vi "Obtain Motor Communication.vi"(8 "error in (no error)":errorcluster, 11 "motor name":string) -> (0 "error out":errorcluster, 1 "found?":bool, 3 "motor communication out":refnum<class "NI_Robotics_Motor Communication.lvclass">)   [LabVIEW 2017, in "NI_Robotics_Motor Communication.lvclass"]
doc: "Obtains and existing communication session for a motor."
uses:
  <vilib>/robotics/Actuation/Motor Communication/NI_Robotics_Motor Communication.lvclass
  <vilib>/robotics/Actuation/Motor Communication/FG Motor Comm Sessions Action.ctl
  <vilib>/robotics/Utilities/Generate Error.vi
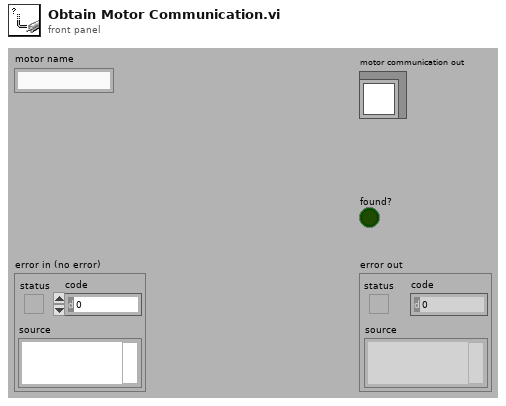
[diagram p1: front panel]
types:
  T1 = typedef "NI_Robotics_Motor Communication.lvclass/FG Motor Comm Sessions Action.ctl" = enum16{"Get", "Add", "Delete"}
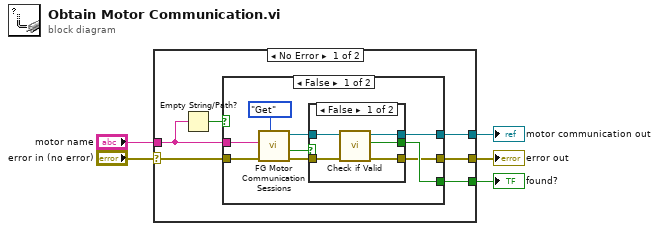
[diagram p0: block diagram]
diagram:
  n1 = case shown="No Error" "error in (no error)" {
    selector: "error in (no error)" -> [w11 w29]
    tunnel: [w9 w29] -> w4
    tunnel: [w8 _] -> w3
    tunnel: "motor name" -> [w7 _]
    tunnel: [w10 _] -> w1
    frame No Error {
      n2 = Empty String/Path?(string/path=w7) -> (empty?=w6:bool)
      n3 = case shown="False" w6 {
        tunnel: w11 -> [w19 w28]
        tunnel: [w15 _] -> w10
        tunnel: [w14 w28] -> w9
        tunnel: [w13 _] -> w8
        tunnel: w7 -> [w12 _]
        frame False {
          n4 = call <vilib>:"FG Motor Communication Sessions.vi"("action"=FG_Motor_Comm_Sessions_Action."Get", "error in (no error)"=w19, "motor name"=w12) -> ("error out"=w18:errorcluster, "failed?"=w16:bool, "motor communication out"=w17:refnum<class "NI_Robotics_Motor Communication.lvclass">)  [unwired: 6 in]
          n5 = case shown="False" w16 {
            tunnel: w17 -> [w25 w26]
            tunnel: [w24 w26] -> w13
            tunnel: w18 -> [w23 w27]
            tunnel: [w21 _] -> w15
            tunnel: [w22 w27] -> w14
            frame False {
              n6 = call <vilib>:"Check if Valid.vi"("error in (no error)"=w23, "motor communication in"=w25) -> ("error out"=w22:errorcluster, "valid?"=w21:bool, "motor communication out"=w24:refnum<class "NI_Robotics_Motor Communication.lvclass">)  [unwired: 7 in]
            }
            frame True {
            }
          }
        }
        frame True {
        }
      }
    }
    frame Error {
    }
  }
  "error out" <- w4
  "motor communication out" <- w3
  "found?" <- w1
